vi "Experiment 17.vi"() -> ()   [LabVIEW 2026]
doc: "Experiment 17\nThis experiment is like Experiment 12 but uses while loops instead of for loops."
uses:
  <vilib>/AdvancedString/1D String Array to Delimited String (string).vi
  <vilib>/Analysis/baseanly.llb/Mean (DBL).vi
  <vilib>/Analysis/NI_AALBase.lvlib
panel:
  out "No. Of Iterations As Block Of Text (easy to copy into Excel)":string
  out "No. Of Iterations Executed - Loop 10":i32
  out "Output - Loop 10":dbl[](array[numeric]) format="%.3f"
  out "No. Of Iterations Executed - Loop 9":i32
  out "Output - Loop 9":dbl[](array[numeric]) format="%.3f"
  out "No. Of Iterations Executed - Loop 8":i32
  out "Output - Loop 8":dbl[](array[numeric]) format="%.3f"
  out "No. Of Iterations Executed - Loop 7":i32
  out "Output - Loop 7":dbl[](array[numeric]) format="%.3f"
  out "No. Of Iterations Executed - Loop 6":i32
  out "Output - Loop 6":dbl[](array[numeric]) format="%.3f"
  out "No. Of Iterations Executed - Loop 5":i32
  out "Output - Loop 5":dbl[](array[numeric]) format="%.3f"
  out "No. Of Iterations Executed - Loop 4":i32
  out "Output - Loop 4":dbl[](array[numeric]) format="%.3f"
  out "No. Of Iterations Executed - Loop 3":i32
  out "Output - Loop 3":dbl[](array[numeric]) format="%.3f"
  out "Avg. No. Of Iterations Executed - All Loops":dbl format="%.1f"
  out "No. Of Iterations Executed - Loop 2":i32
  out "Output - Loop 2":dbl[](array[numeric]) format="%.3f"
  out "No. Of Iterations Executed - Loop 1":i32
  out "Output - Loop 1":dbl[](array[numeric]) format="%.3f"
  out "Stop VI?":bool
  # "Experiment 17"
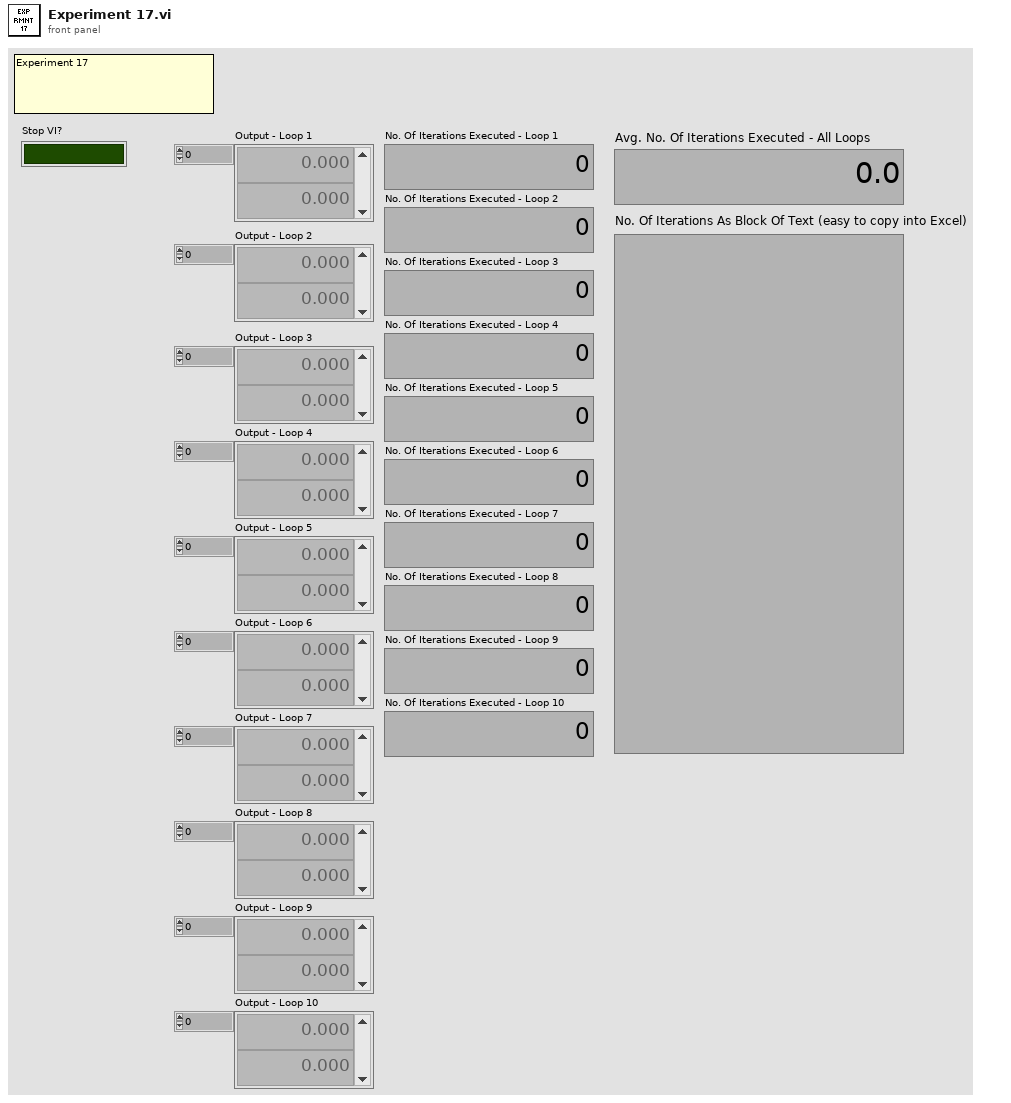
[diagram p1: front panel]
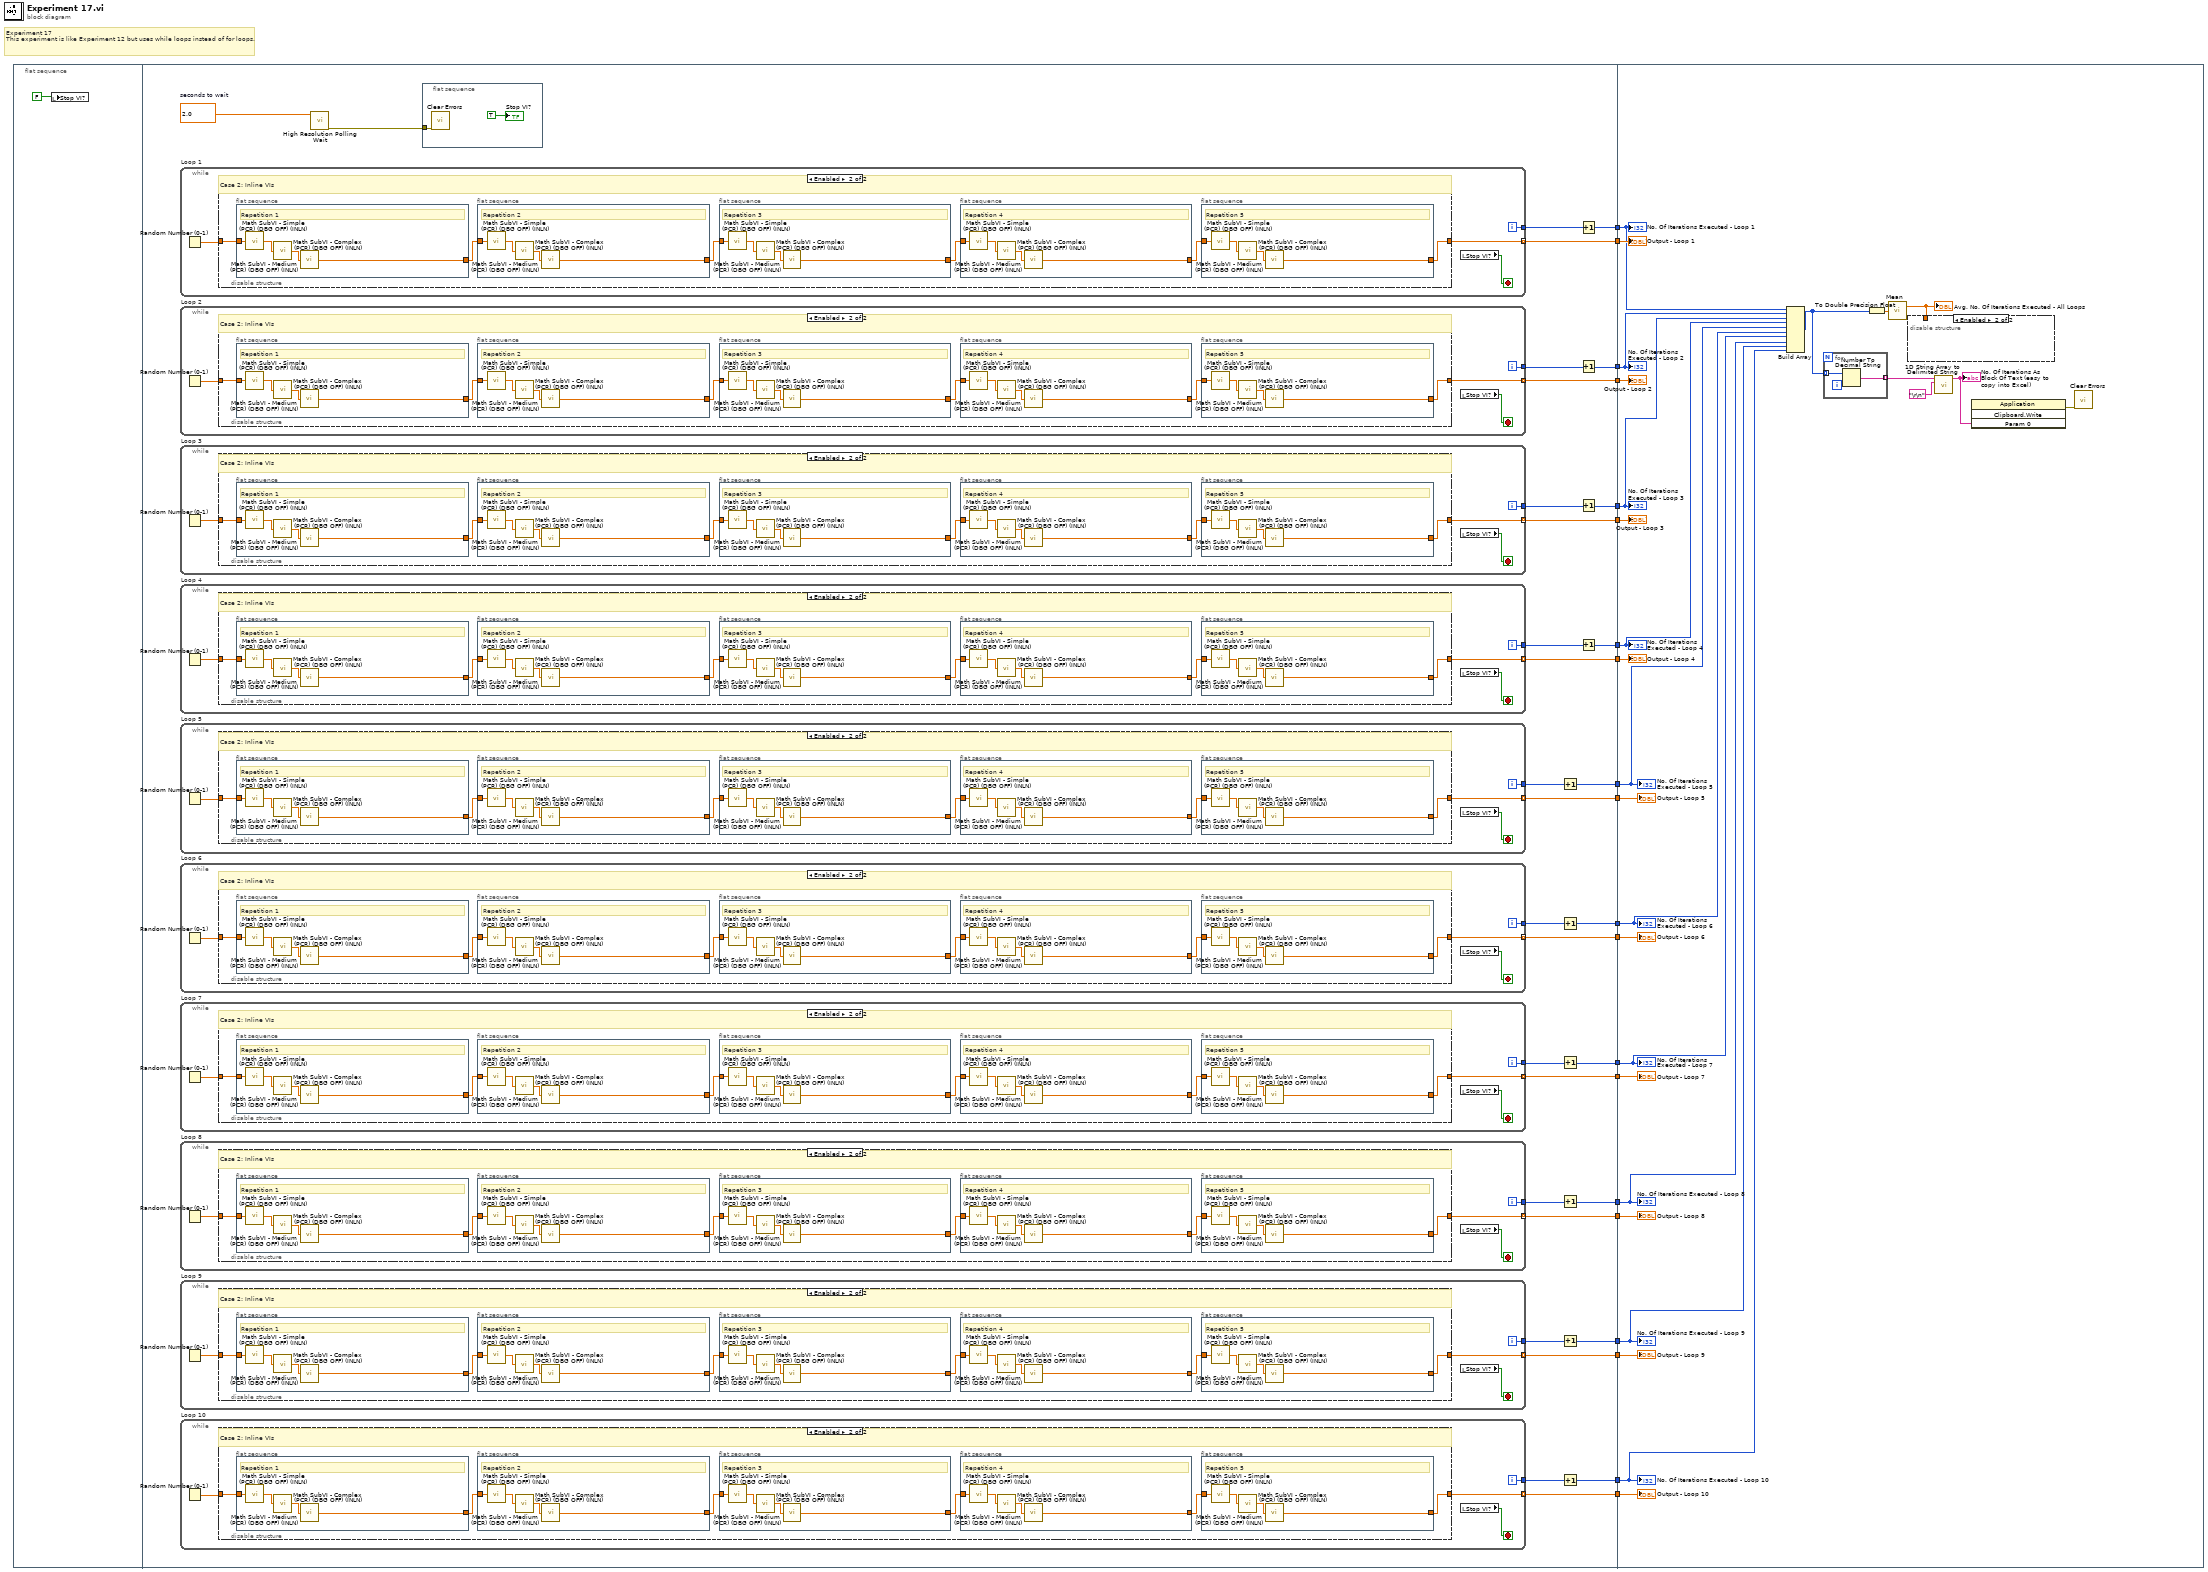
[diagram p0: block diagram]
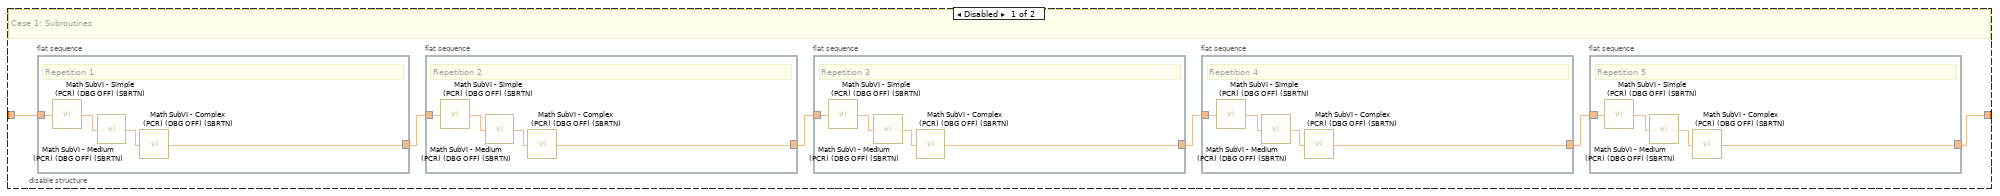
[diagram p2: hidden frame]
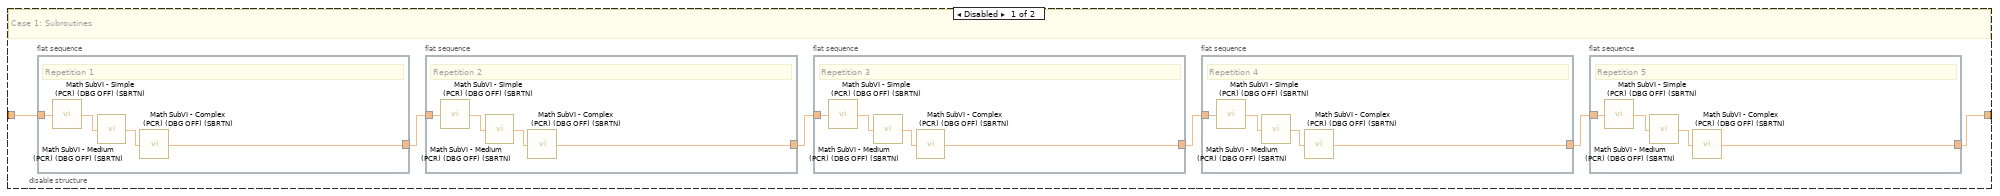
[diagram p3: hidden frame]
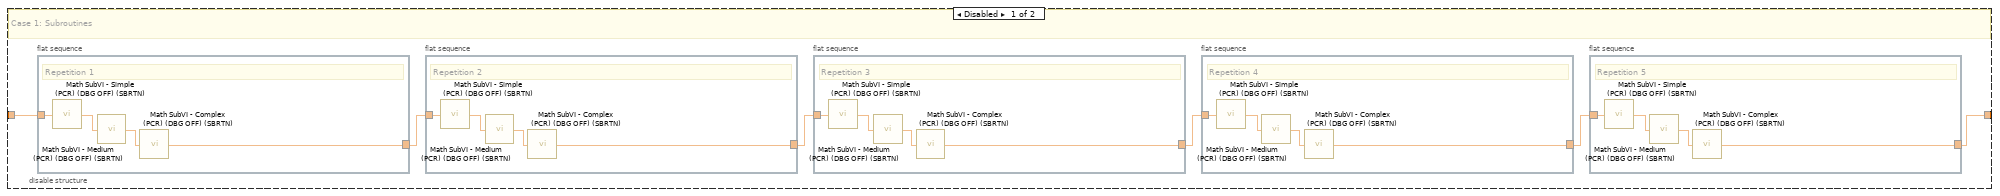
[diagram p4: hidden frame]
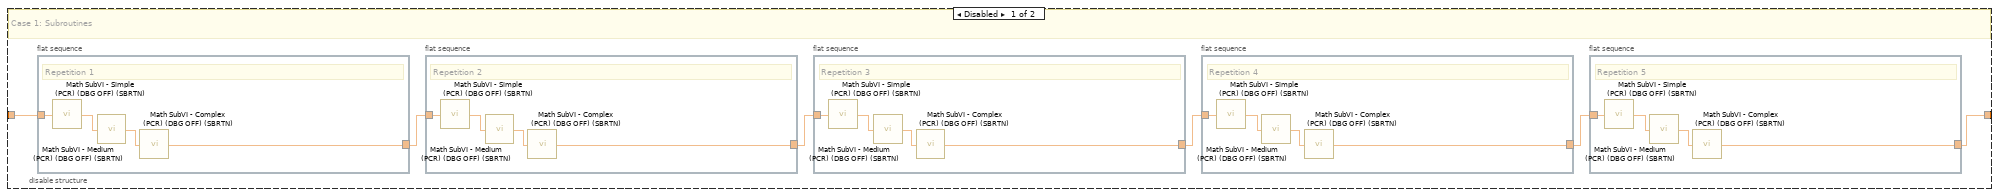
[diagram p5: hidden frame]
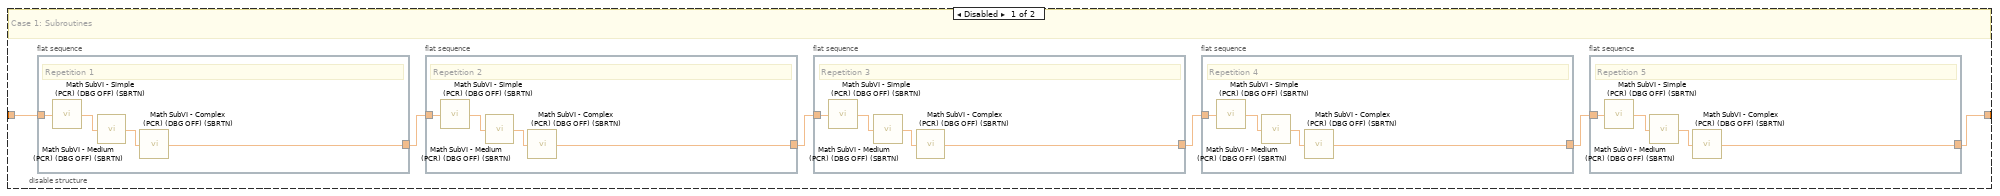
[diagram p6: hidden frame]
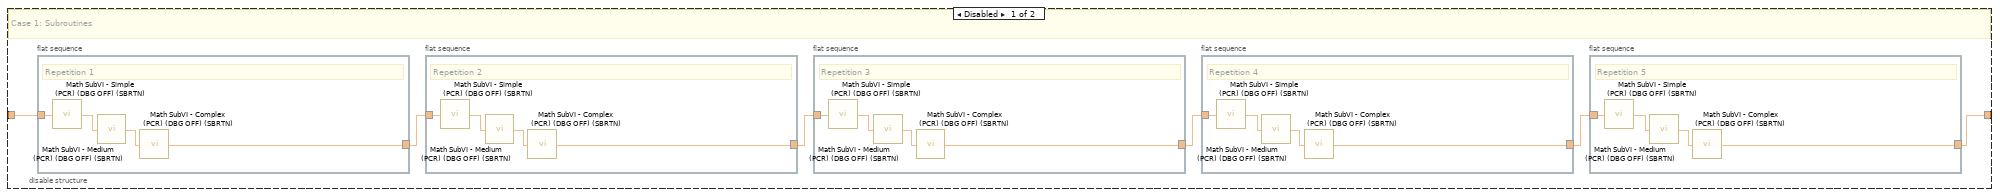
[diagram p7: hidden frame]
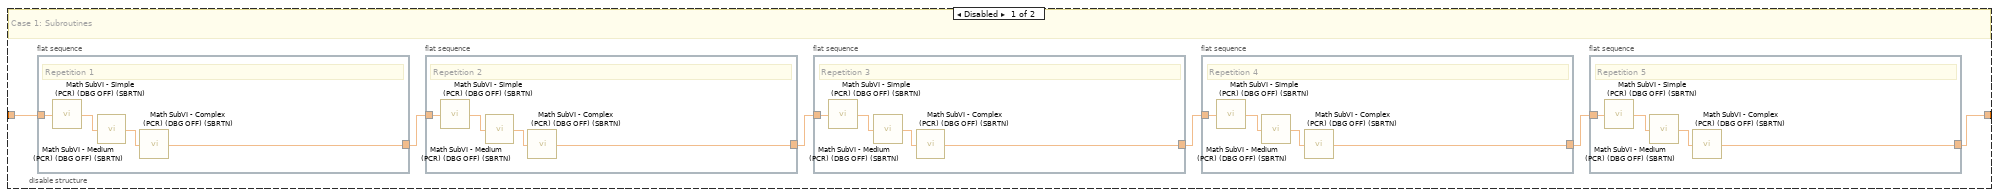
[diagram p8: hidden frame]
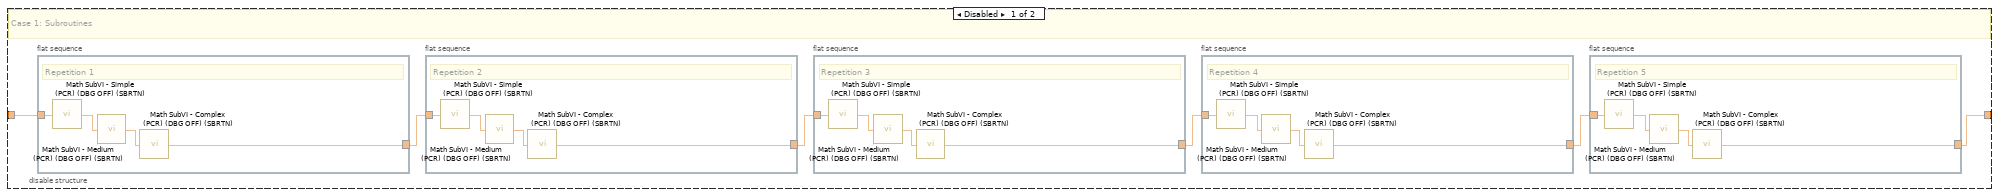
[diagram p9: hidden frame]
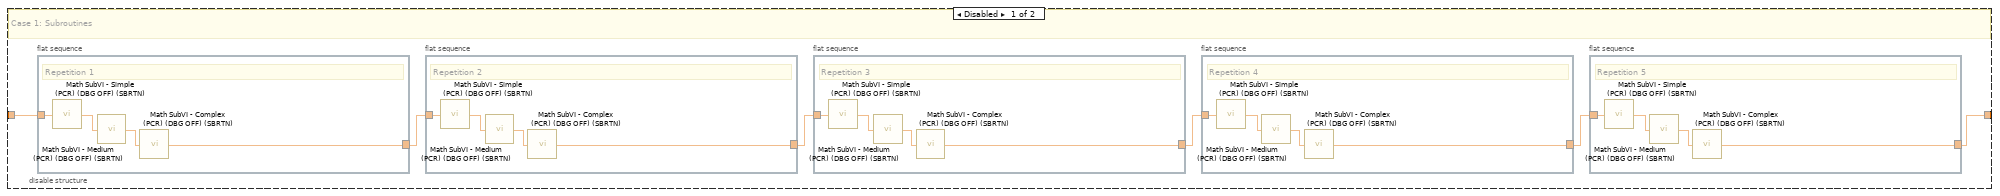
[diagram p10: hidden frame]
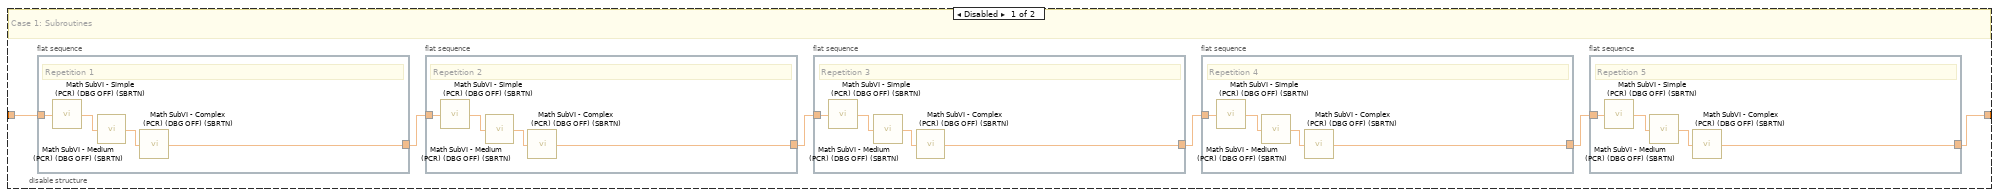
[diagram p11: hidden frame]
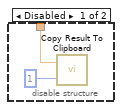
[diagram p12: hidden frame]
diagram:
  # "Experiment 17\nThis experiment is like Experiment 12 but uses while loops instead of for loops."
  n1 = flat-sequence {
    tunnel: [w51] -> w20
    tunnel: [w49] -> w19
    tunnel: [w48] -> w18
    tunnel: [w39] -> w17
    tunnel: [w47] -> w16
    tunnel: [w37] -> w15
    tunnel: [w35] -> w14
    tunnel: [w46] -> w13
    tunnel: [w33] -> w12
    tunnel: [w45] -> w11
    tunnel: [w31] -> w10
    tunnel: [w40] -> w9
    tunnel: [w29] -> w8
    tunnel: [w41] -> w7
    tunnel: [w26] -> w6
    tunnel: [w42] -> w5
    tunnel: [w24] -> w4
    tunnel: [w43] -> w3
    tunnel: [w22] -> w2
    tunnel: [w44] -> w1
    tunnel: w20 -> [w642]
    tunnel: w19 -> [w640]
    tunnel: w18 -> [w639]
    tunnel: w17 -> [w641]
    tunnel: w16 -> [w635]
    tunnel: w15 -> [w637]
    tunnel: w14 -> [w636]
    tunnel: w13 -> [w634]
    tunnel: w12 -> [w632]
    tunnel: w11 -> [w626]
    tunnel: w10 -> [w631]
    tunnel: w9 -> [w625]
    tunnel: w8 -> [w630]
    tunnel: w7 -> [w624]
    tunnel: w6 -> [w629]
    tunnel: w5 -> [w623]
    tunnel: w4 -> [w628]
    tunnel: w3 -> [w622]
    tunnel: w2 -> [w627]
    tunnel: w1 -> [w621]
    frame #0 {
      n2 = local write "Stop VI?"(FALSE) -> ()
    }
    frame #1 {
      w53 = 2.0  # seconds to wait
      n3 = while "Loop 1" {
        tunnel: [w559] -> w51 mode=indexing
        tunnel: [w560] -> w50
        i -> [w560]
        stop <- w561 stop-if-true
        n4 = Random Number (0-1)() -> (number: 0 to 1=w558:dbl)
        n5 = disable-structure shown="Enabled" {
          disable-tunnel: w558 -> [w567 w593]
          disable-tunnel: [w566 w588] -> w559
          frame Disabled {
            # "Case 1: Subroutines"
            n6 = flat-sequence {
              tunnel: w567 -> [w587]
              tunnel: [w584] -> w562
              frame #0 {
                # "Repetition 1"
                n7 = call "Math SubVI - Simple (PCR) (DBG OFF) (SBRTN).vi"("Input"=w587) -> ("Output"=w585:dbl)
                n8 = call "Math SubVI - Medium (PCR) (DBG OFF) (SBRTN).vi"("Input"=w585) -> ("Output"=w586:dbl)
                n9 = call "Math SubVI - Complex (PCR) (DBG OFF) (SBRTN).vi"("Input"=w586) -> ("Output"=w584:dbl)
              }
            }
            n10 = flat-sequence {
              tunnel: w562 -> [w583]
              tunnel: [w580] -> w565
              frame #0 {
                # "Repetition 2"
                n11 = call "Math SubVI - Simple (PCR) (DBG OFF) (SBRTN).vi"("Input"=w583) -> ("Output"=w581:dbl)
                n12 = call "Math SubVI - Medium (PCR) (DBG OFF) (SBRTN).vi"("Input"=w581) -> ("Output"=w582:dbl)
                n13 = call "Math SubVI - Complex (PCR) (DBG OFF) (SBRTN).vi"("Input"=w582) -> ("Output"=w580:dbl)
              }
            }
            n14 = flat-sequence {
              tunnel: w565 -> [w579]
              tunnel: [w576] -> w564
              frame #0 {
                # "Repetition 3"
                n15 = call "Math SubVI - Simple (PCR) (DBG OFF) (SBRTN).vi"("Input"=w579) -> ("Output"=w577:dbl)
                n16 = call "Math SubVI - Medium (PCR) (DBG OFF) (SBRTN).vi"("Input"=w577) -> ("Output"=w578:dbl)
                n17 = call "Math SubVI - Complex (PCR) (DBG OFF) (SBRTN).vi"("Input"=w578) -> ("Output"=w576:dbl)
              }
            }
            n18 = flat-sequence {
              tunnel: w564 -> [w575]
              tunnel: [w572] -> w563
              frame #0 {
                # "Repetition 4"
                n19 = call "Math SubVI - Simple (PCR) (DBG OFF) (SBRTN).vi"("Input"=w575) -> ("Output"=w573:dbl)
                n20 = call "Math SubVI - Medium (PCR) (DBG OFF) (SBRTN).vi"("Input"=w573) -> ("Output"=w574:dbl)
                n21 = call "Math SubVI - Complex (PCR) (DBG OFF) (SBRTN).vi"("Input"=w574) -> ("Output"=w572:dbl)
              }
            }
            n22 = flat-sequence {
              tunnel: w563 -> [w571]
              tunnel: [w568] -> w566
              frame #0 {
                # "Repetition 5"
                n23 = call "Math SubVI - Simple (PCR) (DBG OFF) (SBRTN).vi"("Input"=w571) -> ("Output"=w569:dbl)
                n24 = call "Math SubVI - Medium (PCR) (DBG OFF) (SBRTN).vi"("Input"=w569) -> ("Output"=w570:dbl)
                n25 = call "Math SubVI - Complex (PCR) (DBG OFF) (SBRTN).vi"("Input"=w570) -> ("Output"=w568:dbl)
              }
            }
          }
          frame Enabled {
            # "Case 2: Inline VIs"
            n26 = flat-sequence {
              tunnel: w593 -> [w613]
              tunnel: [w610] -> w592
              frame #0 {
                # "Repetition 1"
                n27 = call "Math SubVI - Simple (PCR) (DBG OFF) (INLN).vi"("Input"=w613) -> ("Output"=w611:dbl)
                n28 = call "Math SubVI - Medium (PCR) (DBG OFF) (INLN).vi"("Input"=w611) -> ("Output"=w612:dbl)
                n29 = call "Math SubVI - Complex (PCR) (DBG OFF) (INLN).vi"("Input"=w612) -> ("Output"=w610:dbl)
              }
            }
            n30 = flat-sequence {
              tunnel: w592 -> [w609]
              tunnel: [w606] -> w591
              frame #0 {
                # "Repetition 2"
                n31 = call "Math SubVI - Simple (PCR) (DBG OFF) (INLN).vi"("Input"=w609) -> ("Output"=w607:dbl)
                n32 = call "Math SubVI - Medium (PCR) (DBG OFF) (INLN).vi"("Input"=w607) -> ("Output"=w608:dbl)
                n33 = call "Math SubVI - Complex (PCR) (DBG OFF) (INLN).vi"("Input"=w608) -> ("Output"=w606:dbl)
              }
            }
            n34 = flat-sequence {
              tunnel: w591 -> [w605]
              tunnel: [w602] -> w590
              frame #0 {
                # "Repetition 3"
                n35 = call "Math SubVI - Simple (PCR) (DBG OFF) (INLN).vi"("Input"=w605) -> ("Output"=w603:dbl)
                n36 = call "Math SubVI - Medium (PCR) (DBG OFF) (INLN).vi"("Input"=w603) -> ("Output"=w604:dbl)
                n37 = call "Math SubVI - Complex (PCR) (DBG OFF) (INLN).vi"("Input"=w604) -> ("Output"=w602:dbl)
              }
            }
            n38 = flat-sequence {
              tunnel: w590 -> [w601]
              tunnel: [w598] -> w589
              frame #0 {
                # "Repetition 4"
                n39 = call "Math SubVI - Simple (PCR) (DBG OFF) (INLN).vi"("Input"=w601) -> ("Output"=w599:dbl)
                n40 = call "Math SubVI - Medium (PCR) (DBG OFF) (INLN).vi"("Input"=w599) -> ("Output"=w600:dbl)
                n41 = call "Math SubVI - Complex (PCR) (DBG OFF) (INLN).vi"("Input"=w600) -> ("Output"=w598:dbl)
              }
            }
            n42 = flat-sequence {
              tunnel: w589 -> [w597]
              tunnel: [w594] -> w588
              frame #0 {
                # "Repetition 5"
                n43 = call "Math SubVI - Simple (PCR) (DBG OFF) (INLN).vi"("Input"=w597) -> ("Output"=w595:dbl)
                n44 = call "Math SubVI - Medium (PCR) (DBG OFF) (INLN).vi"("Input"=w595) -> ("Output"=w596:dbl)
                n45 = call "Math SubVI - Complex (PCR) (DBG OFF) (INLN).vi"("Input"=w596) -> ("Output"=w594:dbl)
              }
            }
          }
        }
        n46 = local read "Stop VI?"() -> (w561:bool)
      }
      n47 = while "Loop 2" {
        tunnel: [w503] -> w39 mode=indexing
        tunnel: [w504] -> w38
        i -> [w504]
        stop <- w505 stop-if-true
        n48 = Random Number (0-1)() -> (number: 0 to 1=w502:dbl)
        n49 = disable-structure shown="Enabled" {
          disable-tunnel: w502 -> [w511 w537]
          disable-tunnel: [w510 w532] -> w503
          frame Disabled {
            # "Case 1: Subroutines"
            n50 = flat-sequence {
              tunnel: w511 -> [w531]
              tunnel: [w528] -> w506
              frame #0 {
                # "Repetition 1"
                n51 = call "Math SubVI - Simple (PCR) (DBG OFF) (SBRTN).vi"("Input"=w531) -> ("Output"=w529:dbl)
                n52 = call "Math SubVI - Medium (PCR) (DBG OFF) (SBRTN).vi"("Input"=w529) -> ("Output"=w530:dbl)
                n53 = call "Math SubVI - Complex (PCR) (DBG OFF) (SBRTN).vi"("Input"=w530) -> ("Output"=w528:dbl)
              }
            }
            n54 = flat-sequence {
              tunnel: w506 -> [w527]
              tunnel: [w524] -> w509
              frame #0 {
                # "Repetition 2"
                n55 = call "Math SubVI - Simple (PCR) (DBG OFF) (SBRTN).vi"("Input"=w527) -> ("Output"=w525:dbl)
                n56 = call "Math SubVI - Medium (PCR) (DBG OFF) (SBRTN).vi"("Input"=w525) -> ("Output"=w526:dbl)
                n57 = call "Math SubVI - Complex (PCR) (DBG OFF) (SBRTN).vi"("Input"=w526) -> ("Output"=w524:dbl)
              }
            }
            n58 = flat-sequence {
              tunnel: w509 -> [w523]
              tunnel: [w520] -> w508
              frame #0 {
                # "Repetition 3"
                n59 = call "Math SubVI - Simple (PCR) (DBG OFF) (SBRTN).vi"("Input"=w523) -> ("Output"=w521:dbl)
                n60 = call "Math SubVI - Medium (PCR) (DBG OFF) (SBRTN).vi"("Input"=w521) -> ("Output"=w522:dbl)
                n61 = call "Math SubVI - Complex (PCR) (DBG OFF) (SBRTN).vi"("Input"=w522) -> ("Output"=w520:dbl)
              }
            }
            n62 = flat-sequence {
              tunnel: w508 -> [w519]
              tunnel: [w516] -> w507
              frame #0 {
                # "Repetition 4"
                n63 = call "Math SubVI - Simple (PCR) (DBG OFF) (SBRTN).vi"("Input"=w519) -> ("Output"=w517:dbl)
                n64 = call "Math SubVI - Medium (PCR) (DBG OFF) (SBRTN).vi"("Input"=w517) -> ("Output"=w518:dbl)
                n65 = call "Math SubVI - Complex (PCR) (DBG OFF) (SBRTN).vi"("Input"=w518) -> ("Output"=w516:dbl)
              }
            }
            n66 = flat-sequence {
              tunnel: w507 -> [w515]
              tunnel: [w512] -> w510
              frame #0 {
                # "Repetition 5"
                n67 = call "Math SubVI - Simple (PCR) (DBG OFF) (SBRTN).vi"("Input"=w515) -> ("Output"=w513:dbl)
                n68 = call "Math SubVI - Medium (PCR) (DBG OFF) (SBRTN).vi"("Input"=w513) -> ("Output"=w514:dbl)
                n69 = call "Math SubVI - Complex (PCR) (DBG OFF) (SBRTN).vi"("Input"=w514) -> ("Output"=w512:dbl)
              }
            }
          }
          frame Enabled {
            # "Case 2: Inline VIs"
            n70 = flat-sequence {
              tunnel: w537 -> [w557]
              tunnel: [w554] -> w536
              frame #0 {
                # "Repetition 1"
                n71 = call "Math SubVI - Simple (PCR) (DBG OFF) (INLN).vi"("Input"=w557) -> ("Output"=w555:dbl)
                n72 = call "Math SubVI - Medium (PCR) (DBG OFF) (INLN).vi"("Input"=w555) -> ("Output"=w556:dbl)
                n73 = call "Math SubVI - Complex (PCR) (DBG OFF) (INLN).vi"("Input"=w556) -> ("Output"=w554:dbl)
              }
            }
            n74 = flat-sequence {
              tunnel: w536 -> [w553]
              tunnel: [w550] -> w535
              frame #0 {
                # "Repetition 2"
                n75 = call "Math SubVI - Simple (PCR) (DBG OFF) (INLN).vi"("Input"=w553) -> ("Output"=w551:dbl)
                n76 = call "Math SubVI - Medium (PCR) (DBG OFF) (INLN).vi"("Input"=w551) -> ("Output"=w552:dbl)
                n77 = call "Math SubVI - Complex (PCR) (DBG OFF) (INLN).vi"("Input"=w552) -> ("Output"=w550:dbl)
              }
            }
            n78 = flat-sequence {
              tunnel: w535 -> [w549]
              tunnel: [w546] -> w534
              frame #0 {
                # "Repetition 3"
                n79 = call "Math SubVI - Simple (PCR) (DBG OFF) (INLN).vi"("Input"=w549) -> ("Output"=w547:dbl)
                n80 = call "Math SubVI - Medium (PCR) (DBG OFF) (INLN).vi"("Input"=w547) -> ("Output"=w548:dbl)
                n81 = call "Math SubVI - Complex (PCR) (DBG OFF) (INLN).vi"("Input"=w548) -> ("Output"=w546:dbl)
              }
            }
            n82 = flat-sequence {
              tunnel: w534 -> [w545]
              tunnel: [w542] -> w533
              frame #0 {
                # "Repetition 4"
                n83 = call "Math SubVI - Simple (PCR) (DBG OFF) (INLN).vi"("Input"=w545) -> ("Output"=w543:dbl)
                n84 = call "Math SubVI - Medium (PCR) (DBG OFF) (INLN).vi"("Input"=w543) -> ("Output"=w544:dbl)
                n85 = call "Math SubVI - Complex (PCR) (DBG OFF) (INLN).vi"("Input"=w544) -> ("Output"=w542:dbl)
              }
            }
            n86 = flat-sequence {
              tunnel: w533 -> [w541]
              tunnel: [w538] -> w532
              frame #0 {
                # "Repetition 5"
                n87 = call "Math SubVI - Simple (PCR) (DBG OFF) (INLN).vi"("Input"=w541) -> ("Output"=w539:dbl)
                n88 = call "Math SubVI - Medium (PCR) (DBG OFF) (INLN).vi"("Input"=w539) -> ("Output"=w540:dbl)
                n89 = call "Math SubVI - Complex (PCR) (DBG OFF) (INLN).vi"("Input"=w540) -> ("Output"=w538:dbl)
              }
            }
          }
        }
        n90 = local read "Stop VI?"() -> (w505:bool)
      }
      n91 = while "Loop 3" {
        tunnel: [w447] -> w37 mode=indexing
        tunnel: [w448] -> w36
        i -> [w448]
        stop <- w449 stop-if-true
        n92 = Random Number (0-1)() -> (number: 0 to 1=w446:dbl)
        n93 = disable-structure shown="Enabled" {
          disable-tunnel: w446 -> [w455 w481]
          disable-tunnel: [w454 w476] -> w447
          frame Disabled {
            # "Case 1: Subroutines"
            n94 = flat-sequence {
              tunnel: w455 -> [w475]
              tunnel: [w472] -> w450
              frame #0 {
                # "Repetition 1"
                n95 = call "Math SubVI - Simple (PCR) (DBG OFF) (SBRTN).vi"("Input"=w475) -> ("Output"=w473:dbl)
                n96 = call "Math SubVI - Medium (PCR) (DBG OFF) (SBRTN).vi"("Input"=w473) -> ("Output"=w474:dbl)
                n97 = call "Math SubVI - Complex (PCR) (DBG OFF) (SBRTN).vi"("Input"=w474) -> ("Output"=w472:dbl)
              }
            }
            n98 = flat-sequence {
              tunnel: w450 -> [w471]
              tunnel: [w468] -> w453
              frame #0 {
                # "Repetition 2"
                n99 = call "Math SubVI - Simple (PCR) (DBG OFF) (SBRTN).vi"("Input"=w471) -> ("Output"=w469:dbl)
                n100 = call "Math SubVI - Medium (PCR) (DBG OFF) (SBRTN).vi"("Input"=w469) -> ("Output"=w470:dbl)
                n101 = call "Math SubVI - Complex (PCR) (DBG OFF) (SBRTN).vi"("Input"=w470) -> ("Output"=w468:dbl)
              }
            }
            n102 = flat-sequence {
              tunnel: w453 -> [w467]
              tunnel: [w464] -> w452
              frame #0 {
                # "Repetition 3"
                n103 = call "Math SubVI - Simple (PCR) (DBG OFF) (SBRTN).vi"("Input"=w467) -> ("Output"=w465:dbl)
                n104 = call "Math SubVI - Medium (PCR) (DBG OFF) (SBRTN).vi"("Input"=w465) -> ("Output"=w466:dbl)
                n105 = call "Math SubVI - Complex (PCR) (DBG OFF) (SBRTN).vi"("Input"=w466) -> ("Output"=w464:dbl)
              }
            }
            n106 = flat-sequence {
              tunnel: w452 -> [w463]
              tunnel: [w460] -> w451
              frame #0 {
                # "Repetition 4"
                n107 = call "Math SubVI - Simple (PCR) (DBG OFF) (SBRTN).vi"("Input"=w463) -> ("Output"=w461:dbl)
                n108 = call "Math SubVI - Medium (PCR) (DBG OFF) (SBRTN).vi"("Input"=w461) -> ("Output"=w462:dbl)
                n109 = call "Math SubVI - Complex (PCR) (DBG OFF) (SBRTN).vi"("Input"=w462) -> ("Output"=w460:dbl)
              }
            }
            n110 = flat-sequence {
              tunnel: w451 -> [w459]
              tunnel: [w456] -> w454
              frame #0 {
                # "Repetition 5"
                n111 = call "Math SubVI - Simple (PCR) (DBG OFF) (SBRTN).vi"("Input"=w459) -> ("Output"=w457:dbl)
                n112 = call "Math SubVI - Medium (PCR) (DBG OFF) (SBRTN).vi"("Input"=w457) -> ("Output"=w458:dbl)
                n113 = call "Math SubVI - Complex (PCR) (DBG OFF) (SBRTN).vi"("Input"=w458) -> ("Output"=w456:dbl)
              }
            }
          }
          frame Enabled {
            # "Case 2: Inline VIs"
            n114 = flat-sequence {
              tunnel: w481 -> [w501]
              tunnel: [w498] -> w480
              frame #0 {
                # "Repetition 1"
                n115 = call "Math SubVI - Simple (PCR) (DBG OFF) (INLN).vi"("Input"=w501) -> ("Output"=w499:dbl)
                n116 = call "Math SubVI - Medium (PCR) (DBG OFF) (INLN).vi"("Input"=w499) -> ("Output"=w500:dbl)
                n117 = call "Math SubVI - Complex (PCR) (DBG OFF) (INLN).vi"("Input"=w500) -> ("Output"=w498:dbl)
              }
            }
            n118 = flat-sequence {
              tunnel: w480 -> [w497]
              tunnel: [w494] -> w479
              frame #0 {
                # "Repetition 2"
                n119 = call "Math SubVI - Simple (PCR) (DBG OFF) (INLN).vi"("Input"=w497) -> ("Output"=w495:dbl)
                n120 = call "Math SubVI - Medium (PCR) (DBG OFF) (INLN).vi"("Input"=w495) -> ("Output"=w496:dbl)
                n121 = call "Math SubVI - Complex (PCR) (DBG OFF) (INLN).vi"("Input"=w496) -> ("Output"=w494:dbl)
              }
            }
            n122 = flat-sequence {
              tunnel: w479 -> [w493]
              tunnel: [w490] -> w478
              frame #0 {
                # "Repetition 3"
                n123 = call "Math SubVI - Simple (PCR) (DBG OFF) (INLN).vi"("Input"=w493) -> ("Output"=w491:dbl)
                n124 = call "Math SubVI - Medium (PCR) (DBG OFF) (INLN).vi"("Input"=w491) -> ("Output"=w492:dbl)
                n125 = call "Math SubVI - Complex (PCR) (DBG OFF) (INLN).vi"("Input"=w492) -> ("Output"=w490:dbl)
              }
            }
            n126 = flat-sequence {
              tunnel: w478 -> [w489]
              tunnel: [w486] -> w477
              frame #0 {
                # "Repetition 4"
                n127 = call "Math SubVI - Simple (PCR) (DBG OFF) (INLN).vi"("Input"=w489) -> ("Output"=w487:dbl)
                n128 = call "Math SubVI - Medium (PCR) (DBG OFF) (INLN).vi"("Input"=w487) -> ("Output"=w488:dbl)
                n129 = call "Math SubVI - Complex (PCR) (DBG OFF) (INLN).vi"("Input"=w488) -> ("Output"=w486:dbl)
              }
            }
            n130 = flat-sequence {
              tunnel: w477 -> [w485]
              tunnel: [w482] -> w476
              frame #0 {
                # "Repetition 5"
                n131 = call "Math SubVI - Simple (PCR) (DBG OFF) (INLN).vi"("Input"=w485) -> ("Output"=w483:dbl)
                n132 = call "Math SubVI - Medium (PCR) (DBG OFF) (INLN).vi"("Input"=w483) -> ("Output"=w484:dbl)
                n133 = call "Math SubVI - Complex (PCR) (DBG OFF) (INLN).vi"("Input"=w484) -> ("Output"=w482:dbl)
              }
            }
          }
        }
        n134 = local read "Stop VI?"() -> (w449:bool)
      }
      n135 = while "Loop 4" {
        tunnel: [w391] -> w35 mode=indexing
        tunnel: [w392] -> w34
        i -> [w392]
        stop <- w393 stop-if-true
        n136 = Random Number (0-1)() -> (number: 0 to 1=w390:dbl)
        n137 = disable-structure shown="Enabled" {
          disable-tunnel: w390 -> [w399 w425]
          disable-tunnel: [w398 w420] -> w391
          frame Disabled {
            # "Case 1: Subroutines"
            n138 = flat-sequence {
              tunnel: w399 -> [w419]
              tunnel: [w416] -> w394
              frame #0 {
                # "Repetition 1"
                n139 = call "Math SubVI - Simple (PCR) (DBG OFF) (SBRTN).vi"("Input"=w419) -> ("Output"=w417:dbl)
                n140 = call "Math SubVI - Medium (PCR) (DBG OFF) (SBRTN).vi"("Input"=w417) -> ("Output"=w418:dbl)
                n141 = call "Math SubVI - Complex (PCR) (DBG OFF) (SBRTN).vi"("Input"=w418) -> ("Output"=w416:dbl)
              }
            }
            n142 = flat-sequence {
              tunnel: w394 -> [w415]
              tunnel: [w412] -> w397
              frame #0 {
                # "Repetition 2"
                n143 = call "Math SubVI - Simple (PCR) (DBG OFF) (SBRTN).vi"("Input"=w415) -> ("Output"=w413:dbl)
                n144 = call "Math SubVI - Medium (PCR) (DBG OFF) (SBRTN).vi"("Input"=w413) -> ("Output"=w414:dbl)
                n145 = call "Math SubVI - Complex (PCR) (DBG OFF) (SBRTN).vi"("Input"=w414) -> ("Output"=w412:dbl)
              }
            }
            n146 = flat-sequence {
              tunnel: w397 -> [w411]
              tunnel: [w408] -> w396
              frame #0 {
                # "Repetition 3"
                n147 = call "Math SubVI - Simple (PCR) (DBG OFF) (SBRTN).vi"("Input"=w411) -> ("Output"=w409:dbl)
                n148 = call "Math SubVI - Medium (PCR) (DBG OFF) (SBRTN).vi"("Input"=w409) -> ("Output"=w410:dbl)
                n149 = call "Math SubVI - Complex (PCR) (DBG OFF) (SBRTN).vi"("Input"=w410) -> ("Output"=w408:dbl)
              }
            }
            n150 = flat-sequence {
              tunnel: w396 -> [w407]
              tunnel: [w404] -> w395
              frame #0 {
                # "Repetition 4"
                n151 = call "Math SubVI - Simple (PCR) (DBG OFF) (SBRTN).vi"("Input"=w407) -> ("Output"=w405:dbl)
                n152 = call "Math SubVI - Medium (PCR) (DBG OFF) (SBRTN).vi"("Input"=w405) -> ("Output"=w406:dbl)
                n153 = call "Math SubVI - Complex (PCR) (DBG OFF) (SBRTN).vi"("Input"=w406) -> ("Output"=w404:dbl)
              }
            }
            n154 = flat-sequence {
              tunnel: w395 -> [w403]
              tunnel: [w400] -> w398
              frame #0 {
                # "Repetition 5"
                n155 = call "Math SubVI - Simple (PCR) (DBG OFF) (SBRTN).vi"("Input"=w403) -> ("Output"=w401:dbl)
                n156 = call "Math SubVI - Medium (PCR) (DBG OFF) (SBRTN).vi"("Input"=w401) -> ("Output"=w402:dbl)
                n157 = call "Math SubVI - Complex (PCR) (DBG OFF) (SBRTN).vi"("Input"=w402) -> ("Output"=w400:dbl)
              }
            }
          }
          frame Enabled {
            # "Case 2: Inline VIs"
            n158 = flat-sequence {
              tunnel: w425 -> [w445]
              tunnel: [w442] -> w424
              frame #0 {
                # "Repetition 1"
                n159 = call "Math SubVI - Simple (PCR) (DBG OFF) (INLN).vi"("Input"=w445) -> ("Output"=w443:dbl)
                n160 = call "Math SubVI - Medium (PCR) (DBG OFF) (INLN).vi"("Input"=w443) -> ("Output"=w444:dbl)
                n161 = call "Math SubVI - Complex (PCR) (DBG OFF) (INLN).vi"("Input"=w444) -> ("Output"=w442:dbl)
              }
            }
            n162 = flat-sequence {
              tunnel: w424 -> [w441]
              tunnel: [w438] -> w423
              frame #0 {
                # "Repetition 2"
                n163 = call "Math SubVI - Simple (PCR) (DBG OFF) (INLN).vi"("Input"=w441) -> ("Output"=w439:dbl)
                n164 = call "Math SubVI - Medium (PCR) (DBG OFF) (INLN).vi"("Input"=w439) -> ("Output"=w440:dbl)
                n165 = call "Math SubVI - Complex (PCR) (DBG OFF) (INLN).vi"("Input"=w440) -> ("Output"=w438:dbl)
              }
            }
            n166 = flat-sequence {
              tunnel: w423 -> [w437]
              tunnel: [w434] -> w422
              frame #0 {
                # "Repetition 3"
                n167 = call "Math SubVI - Simple (PCR) (DBG OFF) (INLN).vi"("Input"=w437) -> ("Output"=w435:dbl)
                n168 = call "Math SubVI - Medium (PCR) (DBG OFF) (INLN).vi"("Input"=w435) -> ("Output"=w436:dbl)
                n169 = call "Math SubVI - Complex (PCR) (DBG OFF) (INLN).vi"("Input"=w436) -> ("Output"=w434:dbl)
              }
            }
            n170 = flat-sequence {
              tunnel: w422 -> [w433]
              tunnel: [w430] -> w421
              frame #0 {
                # "Repetition 4"
                n171 = call "Math SubVI - Simple (PCR) (DBG OFF) (INLN).vi"("Input"=w433) -> ("Output"=w431:dbl)
                n172 = call "Math SubVI - Medium (PCR) (DBG OFF) (INLN).vi"("Input"=w431) -> ("Output"=w432:dbl)
                n173 = call "Math SubVI - Complex (PCR) (DBG OFF) (INLN).vi"("Input"=w432) -> ("Output"=w430:dbl)
              }
            }
            n174 = flat-sequence {
              tunnel: w421 -> [w429]
              tunnel: [w426] -> w420
              frame #0 {
                # "Repetition 5"
                n175 = call "Math SubVI - Simple (PCR) (DBG OFF) (INLN).vi"("Input"=w429) -> ("Output"=w427:dbl)
                n176 = call "Math SubVI - Medium (PCR) (DBG OFF) (INLN).vi"("Input"=w427) -> ("Output"=w428:dbl)
                n177 = call "Math SubVI - Complex (PCR) (DBG OFF) (INLN).vi"("Input"=w428) -> ("Output"=w426:dbl)
              }
            }
          }
        }
        n178 = local read "Stop VI?"() -> (w393:bool)
      }
      n179 = while "Loop 5" {
        tunnel: [w335] -> w33 mode=indexing
        tunnel: [w336] -> w32
        i -> [w336]
        stop <- w337 stop-if-true
        n180 = Random Number (0-1)() -> (number: 0 to 1=w334:dbl)
        n181 = disable-structure shown="Enabled" {
          disable-tunnel: w334 -> [w343 w369]
          disable-tunnel: [w342 w364] -> w335
          frame Disabled {
            # "Case 1: Subroutines"
            n182 = flat-sequence {
              tunnel: w343 -> [w363]
              tunnel: [w360] -> w338
              frame #0 {
                # "Repetition 1"
                n183 = call "Math SubVI - Simple (PCR) (DBG OFF) (SBRTN).vi"("Input"=w363) -> ("Output"=w361:dbl)
                n184 = call "Math SubVI - Medium (PCR) (DBG OFF) (SBRTN).vi"("Input"=w361) -> ("Output"=w362:dbl)
                n185 = call "Math SubVI - Complex (PCR) (DBG OFF) (SBRTN).vi"("Input"=w362) -> ("Output"=w360:dbl)
              }
            }
            n186 = flat-sequence {
              tunnel: w338 -> [w359]
              tunnel: [w356] -> w341
              frame #0 {
                # "Repetition 2"
                n187 = call "Math SubVI - Simple (PCR) (DBG OFF) (SBRTN).vi"("Input"=w359) -> ("Output"=w357:dbl)
                n188 = call "Math SubVI - Medium (PCR) (DBG OFF) (SBRTN).vi"("Input"=w357) -> ("Output"=w358:dbl)
                n189 = call "Math SubVI - Complex (PCR) (DBG OFF) (SBRTN).vi"("Input"=w358) -> ("Output"=w356:dbl)
              }
            }
            n190 = flat-sequence {
              tunnel: w341 -> [w355]
              tunnel: [w352] -> w340
              frame #0 {
                # "Repetition 3"
                n191 = call "Math SubVI - Simple (PCR) (DBG OFF) (SBRTN).vi"("Input"=w355) -> ("Output"=w353:dbl)
                n192 = call "Math SubVI - Medium (PCR) (DBG OFF) (SBRTN).vi"("Input"=w353) -> ("Output"=w354:dbl)
                n193 = call "Math SubVI - Complex (PCR) (DBG OFF) (SBRTN).vi"("Input"=w354) -> ("Output"=w352:dbl)
              }
            }
            n194 = flat-sequence {
              tunnel: w340 -> [w351]
              tunnel: [w348] -> w339
              frame #0 {
                # "Repetition 4"
                n195 = call "Math SubVI - Simple (PCR) (DBG OFF) (SBRTN).vi"("Input"=w351) -> ("Output"=w349:dbl)
                n196 = call "Math SubVI - Medium (PCR) (DBG OFF) (SBRTN).vi"("Input"=w349) -> ("Output"=w350:dbl)
                n197 = call "Math SubVI - Complex (PCR) (DBG OFF) (SBRTN).vi"("Input"=w350) -> ("Output"=w348:dbl)
              }
            }
            n198 = flat-sequence {
              tunnel: w339 -> [w347]
              tunnel: [w344] -> w342
              frame #0 {
                # "Repetition 5"
                n199 = call "Math SubVI - Simple (PCR) (DBG OFF) (SBRTN).vi"("Input"=w347) -> ("Output"=w345:dbl)
                n200 = call "Math SubVI - Medium (PCR) (DBG OFF) (SBRTN).vi"("Input"=w345) -> ("Output"=w346:dbl)
                n201 = call "Math SubVI - Complex (PCR) (DBG OFF) (SBRTN).vi"("Input"=w346) -> ("Output"=w344:dbl)
              }
            }
          }
          frame Enabled {
            # "Case 2: Inline VIs"
            n202 = flat-sequence {
              tunnel: w369 -> [w389]
              tunnel: [w386] -> w368
              frame #0 {
                # "Repetition 1"
                n203 = call "Math SubVI - Simple (PCR) (DBG OFF) (INLN).vi"("Input"=w389) -> ("Output"=w387:dbl)
                n204 = call "Math SubVI - Medium (PCR) (DBG OFF) (INLN).vi"("Input"=w387) -> ("Output"=w388:dbl)
                n205 = call "Math SubVI - Complex (PCR) (DBG OFF) (INLN).vi"("Input"=w388) -> ("Output"=w386:dbl)
              }
            }
            n206 = flat-sequence {
              tunnel: w368 -> [w385]
              tunnel: [w382] -> w367
              frame #0 {
                # "Repetition 2"
                n207 = call "Math SubVI - Simple (PCR) (DBG OFF) (INLN).vi"("Input"=w385) -> ("Output"=w383:dbl)
                n208 = call "Math SubVI - Medium (PCR) (DBG OFF) (INLN).vi"("Input"=w383) -> ("Output"=w384:dbl)
                n209 = call "Math SubVI - Complex (PCR) (DBG OFF) (INLN).vi"("Input"=w384) -> ("Output"=w382:dbl)
              }
            }
            n210 = flat-sequence {
              tunnel: w367 -> [w381]
              tunnel: [w378] -> w366
              frame #0 {
                # "Repetition 3"
                n211 = call "Math SubVI - Simple (PCR) (DBG OFF) (INLN).vi"("Input"=w381) -> ("Output"=w379:dbl)
                n212 = call "Math SubVI - Medium (PCR) (DBG OFF) (INLN).vi"("Input"=w379) -> ("Output"=w380:dbl)
                n213 = call "Math SubVI - Complex (PCR) (DBG OFF) (INLN).vi"("Input"=w380) -> ("Output"=w378:dbl)
              }
            }
            n214 = flat-sequence {
              tunnel: w366 -> [w377]
              tunnel: [w374] -> w365
              frame #0 {
                # "Repetition 4"
                n215 = call "Math SubVI - Simple (PCR) (DBG OFF) (INLN).vi"("Input"=w377) -> ("Output"=w375:dbl)
                n216 = call "Math SubVI - Medium (PCR) (DBG OFF) (INLN).vi"("Input"=w375) -> ("Output"=w376:dbl)
                n217 = call "Math SubVI - Complex (PCR) (DBG OFF) (INLN).vi"("Input"=w376) -> ("Output"=w374:dbl)
              }
            }
            n218 = flat-sequence {
              tunnel: w365 -> [w373]
              tunnel: [w370] -> w364
              frame #0 {
                # "Repetition 5"
                n219 = call "Math SubVI - Simple (PCR) (DBG OFF) (INLN).vi"("Input"=w373) -> ("Output"=w371:dbl)
                n220 = call "Math SubVI - Medium (PCR) (DBG OFF) (INLN).vi"("Input"=w371) -> ("Output"=w372:dbl)
                n221 = call "Math SubVI - Complex (PCR) (DBG OFF) (INLN).vi"("Input"=w372) -> ("Output"=w370:dbl)
              }
            }
          }
        }
        n222 = local read "Stop VI?"() -> (w337:bool)
      }
      n223 = while "Loop 6" {
        tunnel: [w279] -> w31 mode=indexing
        tunnel: [w280] -> w30
        i -> [w280]
        stop <- w281 stop-if-true
        n224 = Random Number (0-1)() -> (number: 0 to 1=w278:dbl)
        n225 = disable-structure shown="Enabled" {
          disable-tunnel: w278 -> [w287 w313]
          disable-tunnel: [w286 w308] -> w279
          frame Disabled {
            # "Case 1: Subroutines"
            n226 = flat-sequence {
              tunnel: w287 -> [w307]
              tunnel: [w304] -> w282
              frame #0 {
                # "Repetition 1"
                n227 = call "Math SubVI - Simple (PCR) (DBG OFF) (SBRTN).vi"("Input"=w307) -> ("Output"=w305:dbl)
                n228 = call "Math SubVI - Medium (PCR) (DBG OFF) (SBRTN).vi"("Input"=w305) -> ("Output"=w306:dbl)
                n229 = call "Math SubVI - Complex (PCR) (DBG OFF) (SBRTN).vi"("Input"=w306) -> ("Output"=w304:dbl)
              }
            }
            n230 = flat-sequence {
              tunnel: w282 -> [w303]
              tunnel: [w300] -> w285
              frame #0 {
                # "Repetition 2"
                n231 = call "Math SubVI - Simple (PCR) (DBG OFF) (SBRTN).vi"("Input"=w303) -> ("Output"=w301:dbl)
                n232 = call "Math SubVI - Medium (PCR) (DBG OFF) (SBRTN).vi"("Input"=w301) -> ("Output"=w302:dbl)
                n233 = call "Math SubVI - Complex (PCR) (DBG OFF) (SBRTN).vi"("Input"=w302) -> ("Output"=w300:dbl)
              }
            }
            n234 = flat-sequence {
              tunnel: w285 -> [w299]
              tunnel: [w296] -> w284
              frame #0 {
                # "Repetition 3"
                n235 = call "Math SubVI - Simple (PCR) (DBG OFF) (SBRTN).vi"("Input"=w299) -> ("Output"=w297:dbl)
                n236 = call "Math SubVI - Medium (PCR) (DBG OFF) (SBRTN).vi"("Input"=w297) -> ("Output"=w298:dbl)
                n237 = call "Math SubVI - Complex (PCR) (DBG OFF) (SBRTN).vi"("Input"=w298) -> ("Output"=w296:dbl)
              }
            }
            n238 = flat-sequence {
              tunnel: w284 -> [w295]
              tunnel: [w292] -> w283
              frame #0 {
                # "Repetition 4"
                n239 = call "Math SubVI - Simple (PCR) (DBG OFF) (SBRTN).vi"("Input"=w295) -> ("Output"=w293:dbl)
                n240 = call "Math SubVI - Medium (PCR) (DBG OFF) (SBRTN).vi"("Input"=w293) -> ("Output"=w294:dbl)
                n241 = call "Math SubVI - Complex (PCR) (DBG OFF) (SBRTN).vi"("Input"=w294) -> ("Output"=w292:dbl)
              }
            }
            n242 = flat-sequence {
              tunnel: w283 -> [w291]
              tunnel: [w288] -> w286
              frame #0 {
                # "Repetition 5"
                n243 = call "Math SubVI - Simple (PCR) (DBG OFF) (SBRTN).vi"("Input"=w291) -> ("Output"=w289:dbl)
                n244 = call "Math SubVI - Medium (PCR) (DBG OFF) (SBRTN).vi"("Input"=w289) -> ("Output"=w290:dbl)
                n245 = call "Math SubVI - Complex (PCR) (DBG OFF) (SBRTN).vi"("Input"=w290) -> ("Output"=w288:dbl)
              }
            }
          }
          frame Enabled {
            # "Case 2: Inline VIs"
            n246 = flat-sequence {
              tunnel: w313 -> [w333]
              tunnel: [w330] -> w312
              frame #0 {
                # "Repetition 1"
                n247 = call "Math SubVI - Simple (PCR) (DBG OFF) (INLN).vi"("Input"=w333) -> ("Output"=w331:dbl)
                n248 = call "Math SubVI - Medium (PCR) (DBG OFF) (INLN).vi"("Input"=w331) -> ("Output"=w332:dbl)
                n249 = call "Math SubVI - Complex (PCR) (DBG OFF) (INLN).vi"("Input"=w332) -> ("Output"=w330:dbl)
              }
            }
            n250 = flat-sequence {
              tunnel: w312 -> [w329]
              tunnel: [w326] -> w311
              frame #0 {
                # "Repetition 2"
                n251 = call "Math SubVI - Simple (PCR) (DBG OFF) (INLN).vi"("Input"=w329) -> ("Output"=w327:dbl)
                n252 = call "Math SubVI - Medium (PCR) (DBG OFF) (INLN).vi"("Input"=w327) -> ("Output"=w328:dbl)
                n253 = call "Math SubVI - Complex (PCR) (DBG OFF) (INLN).vi"("Input"=w328) -> ("Output"=w326:dbl)
              }
            }
            n254 = flat-sequence {
              tunnel: w311 -> [w325]
              tunnel: [w322] -> w310
              frame #0 {
                # "Repetition 3"
                n255 = call "Math SubVI - Simple (PCR) (DBG OFF) (INLN).vi"("Input"=w325) -> ("Output"=w323:dbl)
                n256 = call "Math SubVI - Medium (PCR) (DBG OFF) (INLN).vi"("Input"=w323) -> ("Output"=w324:dbl)
                n257 = call "Math SubVI - Complex (PCR) (DBG OFF) (INLN).vi"("Input"=w324) -> ("Output"=w322:dbl)
              }
            }
            n258 = flat-sequence {
              tunnel: w310 -> [w321]
              tunnel: [w318] -> w309
              frame #0 {
                # "Repetition 4"
                n259 = call "Math SubVI - Simple (PCR) (DBG OFF) (INLN).vi"("Input"=w321) -> ("Output"=w319:dbl)
                n260 = call "Math SubVI - Medium (PCR) (DBG OFF) (INLN).vi"("Input"=w319) -> ("Output"=w320:dbl)
                n261 = call "Math SubVI - Complex (PCR) (DBG OFF) (INLN).vi"("Input"=w320) -> ("Output"=w318:dbl)
              }
            }
            n262 = flat-sequence {
              tunnel: w309 -> [w317]
              tunnel: [w314] -> w308
              frame #0 {
                # "Repetition 5"
                n263 = call "Math SubVI - Simple (PCR) (DBG OFF) (INLN).vi"("Input"=w317) -> ("Output"=w315:dbl)
                n264 = call "Math SubVI - Medium (PCR) (DBG OFF) (INLN).vi"("Input"=w315) -> ("Output"=w316:dbl)
                n265 = call "Math SubVI - Complex (PCR) (DBG OFF) (INLN).vi"("Input"=w316) -> ("Output"=w314:dbl)
              }
            }
          }
        }
        n266 = local read "Stop VI?"() -> (w281:bool)
      }
      n267 = while "Loop 7" {
        tunnel: [w223] -> w29 mode=indexing
        tunnel: [w224] -> w28
        i -> [w224]
        stop <- w225 stop-if-true
        n268 = Random Number (0-1)() -> (number: 0 to 1=w222:dbl)
        n269 = disable-structure shown="Enabled" {
          disable-tunnel: w222 -> [w231 w257]
          disable-tunnel: [w230 w252] -> w223
          frame Disabled {
            # "Case 1: Subroutines"
            n270 = flat-sequence {
              tunnel: w231 -> [w251]
              tunnel: [w248] -> w226
              frame #0 {
                # "Repetition 1"
                n271 = call "Math SubVI - Simple (PCR) (DBG OFF) (SBRTN).vi"("Input"=w251) -> ("Output"=w249:dbl)
                n272 = call "Math SubVI - Medium (PCR) (DBG OFF) (SBRTN).vi"("Input"=w249) -> ("Output"=w250:dbl)
                n273 = call "Math SubVI - Complex (PCR) (DBG OFF) (SBRTN).vi"("Input"=w250) -> ("Output"=w248:dbl)
              }
            }
            n274 = flat-sequence {
              tunnel: w226 -> [w247]
              tunnel: [w244] -> w229
              frame #0 {
                # "Repetition 2"
                n275 = call "Math SubVI - Simple (PCR) (DBG OFF) (SBRTN).vi"("Input"=w247) -> ("Output"=w245:dbl)
                n276 = call "Math SubVI - Medium (PCR) (DBG OFF) (SBRTN).vi"("Input"=w245) -> ("Output"=w246:dbl)
                n277 = call "Math SubVI - Complex (PCR) (DBG OFF) (SBRTN).vi"("Input"=w246) -> ("Output"=w244:dbl)
              }
            }
            n278 = flat-sequence {
              tunnel: w229 -> [w243]
              tunnel: [w240] -> w228
              frame #0 {
                # "Repetition 3"
                n279 = call "Math SubVI - Simple (PCR) (DBG OFF) (SBRTN).vi"("Input"=w243) -> ("Output"=w241:dbl)
                n280 = call "Math SubVI - Medium (PCR) (DBG OFF) (SBRTN).vi"("Input"=w241) -> ("Output"=w242:dbl)
                n281 = call "Math SubVI - Complex (PCR) (DBG OFF) (SBRTN).vi"("Input"=w242) -> ("Output"=w240:dbl)
              }
            }
            n282 = flat-sequence {
              tunnel: w228 -> [w239]
              tunnel: [w236] -> w227
              frame #0 {
                # "Repetition 4"
                n283 = call "Math SubVI - Simple (PCR) (DBG OFF) (SBRTN).vi"("Input"=w239) -> ("Output"=w237:dbl)
                n284 = call "Math SubVI - Medium (PCR) (DBG OFF) (SBRTN).vi"("Input"=w237) -> ("Output"=w238:dbl)
                n285 = call "Math SubVI - Complex (PCR) (DBG OFF) (SBRTN).vi"("Input"=w238) -> ("Output"=w236:dbl)
              }
            }
            n286 = flat-sequence {
              tunnel: w227 -> [w235]
              tunnel: [w232] -> w230
              frame #0 {
                # "Repetition 5"
                n287 = call "Math SubVI - Simple (PCR) (DBG OFF) (SBRTN).vi"("Input"=w235) -> ("Output"=w233:dbl)
                n288 = call "Math SubVI - Medium (PCR) (DBG OFF) (SBRTN).vi"("Input"=w233) -> ("Output"=w234:dbl)
                n289 = call "Math SubVI - Complex (PCR) (DBG OFF) (SBRTN).vi"("Input"=w234) -> ("Output"=w232:dbl)
              }
            }
          }
          frame Enabled {
            # "Case 2: Inline VIs"
            n290 = flat-sequence {
              tunnel: w257 -> [w277]
              tunnel: [w274] -> w256
              frame #0 {
                # "Repetition 1"
                n291 = call "Math SubVI - Simple (PCR) (DBG OFF) (INLN).vi"("Input"=w277) -> ("Output"=w275:dbl)
                n292 = call "Math SubVI - Medium (PCR) (DBG OFF) (INLN).vi"("Input"=w275) -> ("Output"=w276:dbl)
                n293 = call "Math SubVI - Complex (PCR) (DBG OFF) (INLN).vi"("Input"=w276) -> ("Output"=w274:dbl)
              }
            }
            n294 = flat-sequence {
              tunnel: w256 -> [w273]
              tunnel: [w270] -> w255
              frame #0 {
                # "Repetition 2"
                n295 = call "Math SubVI - Simple (PCR) (DBG OFF) (INLN).vi"("Input"=w273) -> ("Output"=w271:dbl)
                n296 = call "Math SubVI - Medium (PCR) (DBG OFF) (INLN).vi"("Input"=w271) -> ("Output"=w272:dbl)
                n297 = call "Math SubVI - Complex (PCR) (DBG OFF) (INLN).vi"("Input"=w272) -> ("Output"=w270:dbl)
              }
            }
            n298 = flat-sequence {
              tunnel: w255 -> [w269]
              tunnel: [w266] -> w254
              frame #0 {
                # "Repetition 3"
                n299 = call "Math SubVI - Simple (PCR) (DBG OFF) (INLN).vi"("Input"=w269) -> ("Output"=w267:dbl)
                n300 = call "Math SubVI - Medium (PCR) (DBG OFF) (INLN).vi"("Input"=w267) -> ("Output"=w268:dbl)
                n301 = call "Math SubVI - Complex (PCR) (DBG OFF) (INLN).vi"("Input"=w268) -> ("Output"=w266:dbl)
              }
            }
            n302 = flat-sequence {
              tunnel: w254 -> [w265]
              tunnel: [w262] -> w253
              frame #0 {
                # "Repetition 4"
                n303 = call "Math SubVI - Simple (PCR) (DBG OFF) (INLN).vi"("Input"=w265) -> ("Output"=w263:dbl)
                n304 = call "Math SubVI - Medium (PCR) (DBG OFF) (INLN).vi"("Input"=w263) -> ("Output"=w264:dbl)
                n305 = call "Math SubVI - Complex (PCR) (DBG OFF) (INLN).vi"("Input"=w264) -> ("Output"=w262:dbl)
              }
            }
            n306 = flat-sequence {
              tunnel: w253 -> [w261]
              tunnel: [w258] -> w252
              frame #0 {
                # "Repetition 5"
                n307 = call "Math SubVI - Simple (PCR) (DBG OFF) (INLN).vi"("Input"=w261) -> ("Output"=w259:dbl)
                n308 = call "Math SubVI - Medium (PCR) (DBG OFF) (INLN).vi"("Input"=w259) -> ("Output"=w260:dbl)
                n309 = call "Math SubVI - Complex (PCR) (DBG OFF) (INLN).vi"("Input"=w260) -> ("Output"=w258:dbl)
              }
            }
          }
        }
        n310 = local read "Stop VI?"() -> (w225:bool)
      }
      n311 = while "Loop 8" {
        tunnel: [w167] -> w26 mode=indexing
        tunnel: [w168] -> w27
        i -> [w168]
        stop <- w169 stop-if-true
        n312 = Random Number (0-1)() -> (number: 0 to 1=w166:dbl)
        n313 = disable-structure shown="Enabled" {
          disable-tunnel: w166 -> [w175 w201]
          disable-tunnel: [w174 w196] -> w167
          frame Disabled {
            # "Case 1: Subroutines"
            n314 = flat-sequence {
              tunnel: w175 -> [w195]
              tunnel: [w192] -> w170
              frame #0 {
                # "Repetition 1"
                n315 = call "Math SubVI - Simple (PCR) (DBG OFF) (SBRTN).vi"("Input"=w195) -> ("Output"=w193:dbl)
                n316 = call "Math SubVI - Medium (PCR) (DBG OFF) (SBRTN).vi"("Input"=w193) -> ("Output"=w194:dbl)
                n317 = call "Math SubVI - Complex (PCR) (DBG OFF) (SBRTN).vi"("Input"=w194) -> ("Output"=w192:dbl)
              }
            }
            n318 = flat-sequence {
              tunnel: w170 -> [w191]
              tunnel: [w188] -> w173
              frame #0 {
                # "Repetition 2"
                n319 = call "Math SubVI - Simple (PCR) (DBG OFF) (SBRTN).vi"("Input"=w191) -> ("Output"=w189:dbl)
                n320 = call "Math SubVI - Medium (PCR) (DBG OFF) (SBRTN).vi"("Input"=w189) -> ("Output"=w190:dbl)
                n321 = call "Math SubVI - Complex (PCR) (DBG OFF) (SBRTN).vi"("Input"=w190) -> ("Output"=w188:dbl)
              }
            }
            n322 = flat-sequence {
              tunnel: w173 -> [w187]
              tunnel: [w184] -> w172
              frame #0 {
                # "Repetition 3"
                n323 = call "Math SubVI - Simple (PCR) (DBG OFF) (SBRTN).vi"("Input"=w187) -> ("Output"=w185:dbl)
                n324 = call "Math SubVI - Medium (PCR) (DBG OFF) (SBRTN).vi"("Input"=w185) -> ("Output"=w186:dbl)
                n325 = call "Math SubVI - Complex (PCR) (DBG OFF) (SBRTN).vi"("Input"=w186) -> ("Output"=w184:dbl)
              }
            }
            n326 = flat-sequence {
              tunnel: w172 -> [w183]
              tunnel: [w180] -> w171
              frame #0 {
                # "Repetition 4"
                n327 = call "Math SubVI - Simple (PCR) (DBG OFF) (SBRTN).vi"("Input"=w183) -> ("Output"=w181:dbl)
                n328 = call "Math SubVI - Medium (PCR) (DBG OFF) (SBRTN).vi"("Input"=w181) -> ("Output"=w182:dbl)
                n329 = call "Math SubVI - Complex (PCR) (DBG OFF) (SBRTN).vi"("Input"=w182) -> ("Output"=w180:dbl)
              }
            }
            n330 = flat-sequence {
              tunnel: w171 -> [w179]
              tunnel: [w176] -> w174
              frame #0 {
                # "Repetition 5"
                n331 = call "Math SubVI - Simple (PCR) (DBG OFF) (SBRTN).vi"("Input"=w179) -> ("Output"=w177:dbl)
                n332 = call "Math SubVI - Medium (PCR) (DBG OFF) (SBRTN).vi"("Input"=w177) -> ("Output"=w178:dbl)
                n333 = call "Math SubVI - Complex (PCR) (DBG OFF) (SBRTN).vi"("Input"=w178) -> ("Output"=w176:dbl)
              }
            }
          }
          frame Enabled {
            # "Case 2: Inline VIs"
            n334 = flat-sequence {
              tunnel: w201 -> [w221]
              tunnel: [w218] -> w200
              frame #0 {
                # "Repetition 1"
                n335 = call "Math SubVI - Simple (PCR) (DBG OFF) (INLN).vi"("Input"=w221) -> ("Output"=w219:dbl)
                n336 = call "Math SubVI - Medium (PCR) (DBG OFF) (INLN).vi"("Input"=w219) -> ("Output"=w220:dbl)
                n337 = call "Math SubVI - Complex (PCR) (DBG OFF) (INLN).vi"("Input"=w220) -> ("Output"=w218:dbl)
              }
            }
            n338 = flat-sequence {
              tunnel: w200 -> [w217]
              tunnel: [w214] -> w199
              frame #0 {
                # "Repetition 2"
                n339 = call "Math SubVI - Simple (PCR) (DBG OFF) (INLN).vi"("Input"=w217) -> ("Output"=w215:dbl)
                n340 = call "Math SubVI - Medium (PCR) (DBG OFF) (INLN).vi"("Input"=w215) -> ("Output"=w216:dbl)
                n341 = call "Math SubVI - Complex (PCR) (DBG OFF) (INLN).vi"("Input"=w216) -> ("Output"=w214:dbl)
              }
            }
            n342 = flat-sequence {
              tunnel: w199 -> [w213]
              tunnel: [w210] -> w198
              frame #0 {
                # "Repetition 3"
                n343 = call "Math SubVI - Simple (PCR) (DBG OFF) (INLN).vi"("Input"=w213) -> ("Output"=w211:dbl)
                n344 = call "Math SubVI - Medium (PCR) (DBG OFF) (INLN).vi"("Input"=w211) -> ("Output"=w212:dbl)
                n345 = call "Math SubVI - Complex (PCR) (DBG OFF) (INLN).vi"("Input"=w212) -> ("Output"=w210:dbl)
              }
            }
            n346 = flat-sequence {
              tunnel: w198 -> [w209]
              tunnel: [w206] -> w197
              frame #0 {
                # "Repetition 4"
                n347 = call "Math SubVI - Simple (PCR) (DBG OFF) (INLN).vi"("Input"=w209) -> ("Output"=w207:dbl)
                n348 = call "Math SubVI - Medium (PCR) (DBG OFF) (INLN).vi"("Input"=w207) -> ("Output"=w208:dbl)
                n349 = call "Math SubVI - Complex (PCR) (DBG OFF) (INLN).vi"("Input"=w208) -> ("Output"=w206:dbl)
              }
            }
            n350 = flat-sequence {
              tunnel: w197 -> [w205]
              tunnel: [w202] -> w196
              frame #0 {
                # "Repetition 5"
                n351 = call "Math SubVI - Simple (PCR) (DBG OFF) (INLN).vi"("Input"=w205) -> ("Output"=w203:dbl)
                n352 = call "Math SubVI - Medium (PCR) (DBG OFF) (INLN).vi"("Input"=w203) -> ("Output"=w204:dbl)
                n353 = call "Math SubVI - Complex (PCR) (DBG OFF) (INLN).vi"("Input"=w204) -> ("Output"=w202:dbl)
              }
            }
          }
        }
        n354 = local read "Stop VI?"() -> (w169:bool)
      }
      n355 = while "Loop 9" {
        tunnel: [w111] -> w24 mode=indexing
        tunnel: [w112] -> w25
        i -> [w112]
        stop <- w113 stop-if-true
        n356 = Random Number (0-1)() -> (number: 0 to 1=w110:dbl)
        n357 = disable-structure shown="Enabled" {
          disable-tunnel: w110 -> [w119 w145]
          disable-tunnel: [w118 w140] -> w111
          frame Disabled {
            # "Case 1: Subroutines"
            n358 = flat-sequence {
              tunnel: w119 -> [w139]
              tunnel: [w136] -> w114
              frame #0 {
                # "Repetition 1"
                n359 = call "Math SubVI - Simple (PCR) (DBG OFF) (SBRTN).vi"("Input"=w139) -> ("Output"=w137:dbl)
                n360 = call "Math SubVI - Medium (PCR) (DBG OFF) (SBRTN).vi"("Input"=w137) -> ("Output"=w138:dbl)
                n361 = call "Math SubVI - Complex (PCR) (DBG OFF) (SBRTN).vi"("Input"=w138) -> ("Output"=w136:dbl)
              }
            }
            n362 = flat-sequence {
              tunnel: w114 -> [w135]
              tunnel: [w132] -> w117
              frame #0 {
                # "Repetition 2"
                n363 = call "Math SubVI - Simple (PCR) (DBG OFF) (SBRTN).vi"("Input"=w135) -> ("Output"=w133:dbl)
                n364 = call "Math SubVI - Medium (PCR) (DBG OFF) (SBRTN).vi"("Input"=w133) -> ("Output"=w134:dbl)
                n365 = call "Math SubVI - Complex (PCR) (DBG OFF) (SBRTN).vi"("Input"=w134) -> ("Output"=w132:dbl)
              }
            }
            n366 = flat-sequence {
              tunnel: w117 -> [w131]
              tunnel: [w128] -> w116
              frame #0 {
                # "Repetition 3"
                n367 = call "Math SubVI - Simple (PCR) (DBG OFF) (SBRTN).vi"("Input"=w131) -> ("Output"=w129:dbl)
                n368 = call "Math SubVI - Medium (PCR) (DBG OFF) (SBRTN).vi"("Input"=w129) -> ("Output"=w130:dbl)
                n369 = call "Math SubVI - Complex (PCR) (DBG OFF) (SBRTN).vi"("Input"=w130) -> ("Output"=w128:dbl)
              }
            }
            n370 = flat-sequence {
              tunnel: w116 -> [w127]
              tunnel: [w124] -> w115
              frame #0 {
                # "Repetition 4"
                n371 = call "Math SubVI - Simple (PCR) (DBG OFF) (SBRTN).vi"("Input"=w127) -> ("Output"=w125:dbl)
                n372 = call "Math SubVI - Medium (PCR) (DBG OFF) (SBRTN).vi"("Input"=w125) -> ("Output"=w126:dbl)
                n373 = call "Math SubVI - Complex (PCR) (DBG OFF) (SBRTN).vi"("Input"=w126) -> ("Output"=w124:dbl)
              }
            }
            n374 = flat-sequence {
              tunnel: w115 -> [w123]
              tunnel: [w120] -> w118
              frame #0 {
                # "Repetition 5"
                n375 = call "Math SubVI - Simple (PCR) (DBG OFF) (SBRTN).vi"("Input"=w123) -> ("Output"=w121:dbl)
                n376 = call "Math SubVI - Medium (PCR) (DBG OFF) (SBRTN).vi"("Input"=w121) -> ("Output"=w122:dbl)
                n377 = call "Math SubVI - Complex (PCR) (DBG OFF) (SBRTN).vi"("Input"=w122) -> ("Output"=w120:dbl)
              }
            }
          }
          frame Enabled {
            # "Case 2: Inline VIs"
            n378 = flat-sequence {
              tunnel: w145 -> [w165]
              tunnel: [w162] -> w144
              frame #0 {
                # "Repetition 1"
                n379 = call "Math SubVI - Simple (PCR) (DBG OFF) (INLN).vi"("Input"=w165) -> ("Output"=w163:dbl)
                n380 = call "Math SubVI - Medium (PCR) (DBG OFF) (INLN).vi"("Input"=w163) -> ("Output"=w164:dbl)
                n381 = call "Math SubVI - Complex (PCR) (DBG OFF) (INLN).vi"("Input"=w164) -> ("Output"=w162:dbl)
              }
            }
            n382 = flat-sequence {
              tunnel: w144 -> [w161]
              tunnel: [w158] -> w143
              frame #0 {
                # "Repetition 2"
                n383 = call "Math SubVI - Simple (PCR) (DBG OFF) (INLN).vi"("Input"=w161) -> ("Output"=w159:dbl)
                n384 = call "Math SubVI - Medium (PCR) (DBG OFF) (INLN).vi"("Input"=w159) -> ("Output"=w160:dbl)
                n385 = call "Math SubVI - Complex (PCR) (DBG OFF) (INLN).vi"("Input"=w160) -> ("Output"=w158:dbl)
              }
            }
            n386 = flat-sequence {
              tunnel: w143 -> [w157]
              tunnel: [w154] -> w142
              frame #0 {
                # "Repetition 3"
                n387 = call "Math SubVI - Simple (PCR) (DBG OFF) (INLN).vi"("Input"=w157) -> ("Output"=w155:dbl)
                n388 = call "Math SubVI - Medium (PCR) (DBG OFF) (INLN).vi"("Input"=w155) -> ("Output"=w156:dbl)
                n389 = call "Math SubVI - Complex (PCR) (DBG OFF) (INLN).vi"("Input"=w156) -> ("Output"=w154:dbl)
              }
            }
            n390 = flat-sequence {
              tunnel: w142 -> [w153]
              tunnel: [w150] -> w141
              frame #0 {
                # "Repetition 4"
                n391 = call "Math SubVI - Simple (PCR) (DBG OFF) (INLN).vi"("Input"=w153) -> ("Output"=w151:dbl)
                n392 = call "Math SubVI - Medium (PCR) (DBG OFF) (INLN).vi"("Input"=w151) -> ("Output"=w152:dbl)
                n393 = call "Math SubVI - Complex (PCR) (DBG OFF) (INLN).vi"("Input"=w152) -> ("Output"=w150:dbl)
              }
            }
            n394 = flat-sequence {
              tunnel: w141 -> [w149]
              tunnel: [w146] -> w140
              frame #0 {
                # "Repetition 5"
                n395 = call "Math SubVI - Simple (PCR) (DBG OFF) (INLN).vi"("Input"=w149) -> ("Output"=w147:dbl)
                n396 = call "Math SubVI - Medium (PCR) (DBG OFF) (INLN).vi"("Input"=w147) -> ("Output"=w148:dbl)
                n397 = call "Math SubVI - Complex (PCR) (DBG OFF) (INLN).vi"("Input"=w148) -> ("Output"=w146:dbl)
              }
            }
          }
        }
        n398 = local read "Stop VI?"() -> (w113:bool)
      }
      n399 = while "Loop 10" {
        tunnel: [w55] -> w22 mode=indexing
        tunnel: [w56] -> w23
        i -> [w56]
        stop <- w57 stop-if-true
        n400 = Random Number (0-1)() -> (number: 0 to 1=w54:dbl)
        n401 = disable-structure shown="Enabled" {
          disable-tunnel: w54 -> [w63 w89]
          disable-tunnel: [w62 w84] -> w55
          frame Disabled {
            # "Case 1: Subroutines"
            n402 = flat-sequence {
              tunnel: w63 -> [w83]
              tunnel: [w80] -> w58
              frame #0 {
                # "Repetition 1"
                n403 = call "Math SubVI - Simple (PCR) (DBG OFF) (SBRTN).vi"("Input"=w83) -> ("Output"=w81:dbl)
                n404 = call "Math SubVI - Medium (PCR) (DBG OFF) (SBRTN).vi"("Input"=w81) -> ("Output"=w82:dbl)
                n405 = call "Math SubVI - Complex (PCR) (DBG OFF) (SBRTN).vi"("Input"=w82) -> ("Output"=w80:dbl)
              }
            }
            n406 = flat-sequence {
              tunnel: w58 -> [w79]
              tunnel: [w76] -> w61
              frame #0 {
                # "Repetition 2"
                n407 = call "Math SubVI - Simple (PCR) (DBG OFF) (SBRTN).vi"("Input"=w79) -> ("Output"=w77:dbl)
                n408 = call "Math SubVI - Medium (PCR) (DBG OFF) (SBRTN).vi"("Input"=w77) -> ("Output"=w78:dbl)
                n409 = call "Math SubVI - Complex (PCR) (DBG OFF) (SBRTN).vi"("Input"=w78) -> ("Output"=w76:dbl)
              }
            }
            n410 = flat-sequence {
              tunnel: w61 -> [w75]
              tunnel: [w72] -> w60
              frame #0 {
                # "Repetition 3"
                n411 = call "Math SubVI - Simple (PCR) (DBG OFF) (SBRTN).vi"("Input"=w75) -> ("Output"=w73:dbl)
                n412 = call "Math SubVI - Medium (PCR) (DBG OFF) (SBRTN).vi"("Input"=w73) -> ("Output"=w74:dbl)
                n413 = call "Math SubVI - Complex (PCR) (DBG OFF) (SBRTN).vi"("Input"=w74) -> ("Output"=w72:dbl)
              }
            }
            n414 = flat-sequence {
              tunnel: w60 -> [w71]
              tunnel: [w68] -> w59
              frame #0 {
                # "Repetition 4"
                n415 = call "Math SubVI - Simple (PCR) (DBG OFF) (SBRTN).vi"("Input"=w71) -> ("Output"=w69:dbl)
                n416 = call "Math SubVI - Medium (PCR) (DBG OFF) (SBRTN).vi"("Input"=w69) -> ("Output"=w70:dbl)
                n417 = call "Math SubVI - Complex (PCR) (DBG OFF) (SBRTN).vi"("Input"=w70) -> ("Output"=w68:dbl)
              }
            }
            n418 = flat-sequence {
              tunnel: w59 -> [w67]
              tunnel: [w64] -> w62
              frame #0 {
                # "Repetition 5"
                n419 = call "Math SubVI - Simple (PCR) (DBG OFF) (SBRTN).vi"("Input"=w67) -> ("Output"=w65:dbl)
                n420 = call "Math SubVI - Medium (PCR) (DBG OFF) (SBRTN).vi"("Input"=w65) -> ("Output"=w66:dbl)
                n421 = call "Math SubVI - Complex (PCR) (DBG OFF) (SBRTN).vi"("Input"=w66) -> ("Output"=w64:dbl)
              }
            }
          }
          frame Enabled {
            # "Case 2: Inline VIs"
            n422 = flat-sequence {
              tunnel: w89 -> [w109]
              tunnel: [w106] -> w88
              frame #0 {
                # "Repetition 1"
                n423 = call "Math SubVI - Simple (PCR) (DBG OFF) (INLN).vi"("Input"=w109) -> ("Output"=w107:dbl)
                n424 = call "Math SubVI - Medium (PCR) (DBG OFF) (INLN).vi"("Input"=w107) -> ("Output"=w108:dbl)
                n425 = call "Math SubVI - Complex (PCR) (DBG OFF) (INLN).vi"("Input"=w108) -> ("Output"=w106:dbl)
              }
            }
            n426 = flat-sequence {
              tunnel: w88 -> [w105]
              tunnel: [w102] -> w87
              frame #0 {
                # "Repetition 2"
                n427 = call "Math SubVI - Simple (PCR) (DBG OFF) (INLN).vi"("Input"=w105) -> ("Output"=w103:dbl)
                n428 = call "Math SubVI - Medium (PCR) (DBG OFF) (INLN).vi"("Input"=w103) -> ("Output"=w104:dbl)
                n429 = call "Math SubVI - Complex (PCR) (DBG OFF) (INLN).vi"("Input"=w104) -> ("Output"=w102:dbl)
              }
            }
            n430 = flat-sequence {
              tunnel: w87 -> [w101]
              tunnel: [w98] -> w86
              frame #0 {
                # "Repetition 3"
                n431 = call "Math SubVI - Simple (PCR) (DBG OFF) (INLN).vi"("Input"=w101) -> ("Output"=w99:dbl)
                n432 = call "Math SubVI - Medium (PCR) (DBG OFF) (INLN).vi"("Input"=w99) -> ("Output"=w100:dbl)
                n433 = call "Math SubVI - Complex (PCR) (DBG OFF) (INLN).vi"("Input"=w100) -> ("Output"=w98:dbl)
              }
            }
            n434 = flat-sequence {
              tunnel: w86 -> [w97]
              tunnel: [w94] -> w85
              frame #0 {
                # "Repetition 4"
                n435 = call "Math SubVI - Simple (PCR) (DBG OFF) (INLN).vi"("Input"=w97) -> ("Output"=w95:dbl)
                n436 = call "Math SubVI - Medium (PCR) (DBG OFF) (INLN).vi"("Input"=w95) -> ("Output"=w96:dbl)
                n437 = call "Math SubVI - Complex (PCR) (DBG OFF) (INLN).vi"("Input"=w96) -> ("Output"=w94:dbl)
              }
            }
            n438 = flat-sequence {
              tunnel: w85 -> [w93]
              tunnel: [w90] -> w84
              frame #0 {
                # "Repetition 5"
                n439 = call "Math SubVI - Simple (PCR) (DBG OFF) (INLN).vi"("Input"=w93) -> ("Output"=w91:dbl)
                n440 = call "Math SubVI - Medium (PCR) (DBG OFF) (INLN).vi"("Input"=w91) -> ("Output"=w92:dbl)
                n441 = call "Math SubVI - Complex (PCR) (DBG OFF) (INLN).vi"("Input"=w92) -> ("Output"=w90:dbl)
              }
            }
          }
        }
        n442 = local read "Stop VI?"() -> (w57:bool)
      }
      n443 = call <vilib>:"High Resolution Polling Wait.vi"("seconds to wait"=w53) -> ("error out"=w52:errorcluster)  [unwired: 10 in]
      n444 = flat-sequence {
        tunnel: w52 -> [w614]
        frame #0 {
          n445 = call <vilib>:"Clear Errors.vi"("error in (no error)"=w614) -> ()  [unwired: 5 in, 2 out]
          "Stop VI?" <- TRUE
        }
      }
      n446 = Increment(x=w32) -> (x+1=w45:i32)
      n447 = Increment(x=w30) -> (x+1=w40:i32)
      n448 = Increment(x=w28) -> (x+1=w41:i32)
      n449 = Increment(x=w27) -> (x+1=w42:i32)
      n450 = Increment(x=w25) -> (x+1=w43:i32)
      n451 = Increment(x=w23) -> (x+1=w44:i32)
      n452 = Increment(x=w50) -> (x+1=w49:i32)
      n453 = Increment(x=w38) -> (x+1=w48:i32)
      n454 = Increment(x=w36) -> (x+1=w47:i32)
      n455 = Increment(x=w34) -> (x+1=w46:i32)
    }
    frame #2 {
      n456 = Build Array(w640, w639, w635, w634, w626, w625, w624, w623, w622, w621) -> (w620:i32[])
      n457 = for {
        tunnel: w620 -> [w646] mode=indexing
        tunnel: [w645] -> w619 mode=indexing
        n458 = Number To Decimal String(number=w646) -> (decimal integer string=w645:string)  [unwired: 1 in]
      }
      n459 = To Double Precision Float(number=w620) -> (double precision float=w633:dbl[])
      n460 = call-poly <vilib>:"Mean.vi"("X"=w633) -> ("mean"=w638:dbl)  [unwired: 1 out]
      "Avg. No. Of Iterations Executed - All Loops" <- w638
      n461 = disable-structure shown="Enabled" {
        disable-tunnel: w638 -> [w644 _]
        frame Disabled {
          n462 = call "Copy Result To Clipboard.vi"("No. Of Decimal Places (6)"=u32 1, "Input"=w644) -> ()
        }
        frame Enabled {
        }
      }
      n463 = call-poly <vilib>:"1D String Array to Delimited String.vi"("delimiter"="\r\n", "string array"=w619) -> ("delimited string"=w616:string)  [unwired: 9 in]
      "No. Of Iterations As Block Of Text (easy to copy into Excel)" <- w616
      n464 = invoke class="Application" method="Clipboard.Write"("Param 0"=w616) -> (error out=w617:errorcluster)  [unwired: 3 in, 3 out]
      n465 = call <vilib>:"Clear Errors.vi"("error in (no error)"=w617) -> ()  [unwired: 5 in, 2 out]
      "No. Of Iterations Executed - Loop 1" <- w640
      "Output - Loop 1" <- w642
      "No. Of Iterations Executed - Loop 2" <- w639
      "Output - Loop 2" <- w641
      "No. Of Iterations Executed - Loop 3" <- w635
      "Output - Loop 3" <- w637
      "No. Of Iterations Executed - Loop 4" <- w634
      "Output - Loop 4" <- w636
      "No. Of Iterations Executed - Loop 5" <- w626
      "Output - Loop 5" <- w632
      "No. Of Iterations Executed - Loop 6" <- w625
      "Output - Loop 6" <- w631
      "No. Of Iterations Executed - Loop 7" <- w624
      "Output - Loop 7" <- w630
      "No. Of Iterations Executed - Loop 8" <- w623
      "Output - Loop 8" <- w629
      "No. Of Iterations Executed - Loop 9" <- w622
      "Output - Loop 9" <- w628
      "No. Of Iterations Executed - Loop 10" <- w621
      "Output - Loop 10" <- w627
    }
  }
